vi "Controller Test Bench (10) - Output Not Working.vi"() -> ()   [LabVIEW 2022 SP3]
uses:
  WhiteNoise.ctl
  <vilib>/sound2/lvsound2.llb/Sound Data Format.ctl
  <vilib>/Utility/error.llb/DialogType.ctl
  <vilib>/sound2/lvsound2.llb/Sampling Mode.ctl
  <vilib>/sound2/lvsound2.llb/Sound File Refnum.ctl
  <vilib>/Analysis/4window.llb/windowTd.ctl
  <vilib>/DAQmx/write.llb/DAQmx Write (Analog 1D Wfm NChan NSamp).vi
  <vilib>/DAQmx/read.llb/DAQmx Read (Analog 1D Wfm NChan NSamp).vi
  <vilib>/DAQmx/create/channels.llb/DAQmx Create Channel (AO-Voltage-Basic).vi
  <vilib>/DAQmx/create/channels.llb/DAQmx Create Channel (AI-Acceleration-Accelerometer).vi
  <vilib>/DAQmx/configure/timing.llb/DAQmx Timing (Sample Clock).vi
  <vilib>/sound2/lvsound2.llb/Sound File Info (path).vi
  <vilib>/sound2/lvsound2.llb/Sound File Read Open.vi
  <vilib>/DAQmx/configure/task.llb/DAQmx Configure Logging (TDMS).vi
  <vilib>/sound2/lvsound2.llb/Sound File Read (DBL).vi
  <vilib>/DAQmx/miscellaneous.llb/DAQmx Fill In Error Info.vi
  <vilib>/sound2/lvsound2.llb/Sound Output Set Volume (Single).vi
  <vilib>/sound2/lvsound2.llb/Sound Output Write (DBL).vi
  <vilib>/addons/control/pid/pid.llb/PID (DBL Array).vi
  <vilib>/sound2/lvsound2.llb/Sound Output Write (DBL Single).vi
  <vilib>/measure/maspectr.llb/FFT Spectrum (Mag-Phase) for N Chan.vi
  <vilib>/measure/NI_MAPro.lvlib
  <resource>/objmgr/daqmx.rc
  <vilib>/Analysis/NI_AALPro.lvlib
  <vilib>/measure/NI_MABase.lvlib
  <vilib>/addons/control/pid/NI_PID_pid.lvlib
panel:
  in  "Log Data":bool
  in  "Folder to save file to":path=path "C:/Users/LAV-UFSC/OneDrive - UFSC/Documents/LAV - TCC/Dados-Experimentos/Dados Bancada LABVIEW"
  in  "Display Raw Accel. Readings [m/s^2]":bool=TRUE
  in  "Display Output Signal [V]":bool=TRUE
  out "Output Signal":waveform(dbl)[](graph)
  in  "Number of Samples":i32=41200
  in  "Output Noise":bool=TRUE
  in  "?":T1(tab)=enum."Harmonic"
  in  "number of samples/ch (-1: all)":i32=-1
  in  "Path Sound File":path=path "C:/Users/LAV-UFSC-2023/Documents/LAV-TCC/Dados-Experimentos/Dados Empíricos/Uni - vazio.wav"
  in  "Ganho":i32
  in  "Cluster":T3={"Seed"=0.0, "Standard Deviation"=0.2, "Reset"=FALSE, "Iterator"=1.0} {"Standard Deviation" format="%0.2p"}
  in  "Cluster 2":T4={"Iterator"=1.0, "Waveform Type"=0, "Frequency"=10.0, "Amplitude"=0.25} {"Frequency" format="%0.2p"; "Waveform Type" items=["Sine Wave", "Triangle Wave", "Square Wave", "Sawtooth Wave"]; "Amplitude" format="%0.2p"}
  in  "Active Control":bool
  in  "Tab Control":T5(tab)
  in  "reinitialize? (F)":bool
  out "dt out (s)":dbl format="%.3f"
  in  "setpoint":dbl[](array[numeric])=[0.0] format="%.2f"
  in  "PID gains":T6(array[cluster])=[{"proportional gain (Kc)"=1.0, "integral time (Ti, min)"=0.01, "derivative time (Td, min)"=0.0}] {"derivative time (Td, min)" format="%.3f"; "integral time (Ti, min)" format="%.3f"; "proportional gain (Kc)" format="%.3f"}
  in  "dt (s)":dbl=-1.0 format="%.3f"
  in  "output range":cluster{"output high":dbl, "output low":dbl}[](array[cluster])=[{"output high"=100.0, "output low"=-100.0}] {"output low" format="%.2f"; "output high" format="%.2f"}
  in  "Setpoint":dbl
  in  "Gain":dbl min=0.0 step=0.01
  out "Controller Output Signal":waveform(dbl)[](graph)
  in  "Display Output Control Signal [V]":bool
  out "Actual Sample Rate":dbl=1000.0 format="%0.2f"
  out "Accel.1":waveform(dbl)[](graph)
  out "Accel.2":waveform(dbl)[](graph)
  out "Phase 2":cluster{"f0":dbl, "df":dbl, "phase":dbl[]}[](graph)
  out "Mag 2":cluster{"f0":dbl, "df":dbl, "magnitude":dbl[]}[](graph)
  in  "Show FFT":bool=TRUE
  in  "Save FFT":bool
  in  "Start Reading":bool=TRUE
  in  "Stop":bool
  # "Active Controller"
  # "Output Noise"
  # "Data Acquisition"
  # "RAW - Accel. 1"
  # "FFT - Amplitude"
  # "FFT - Phase"
  # "RAW - Accel. 2"
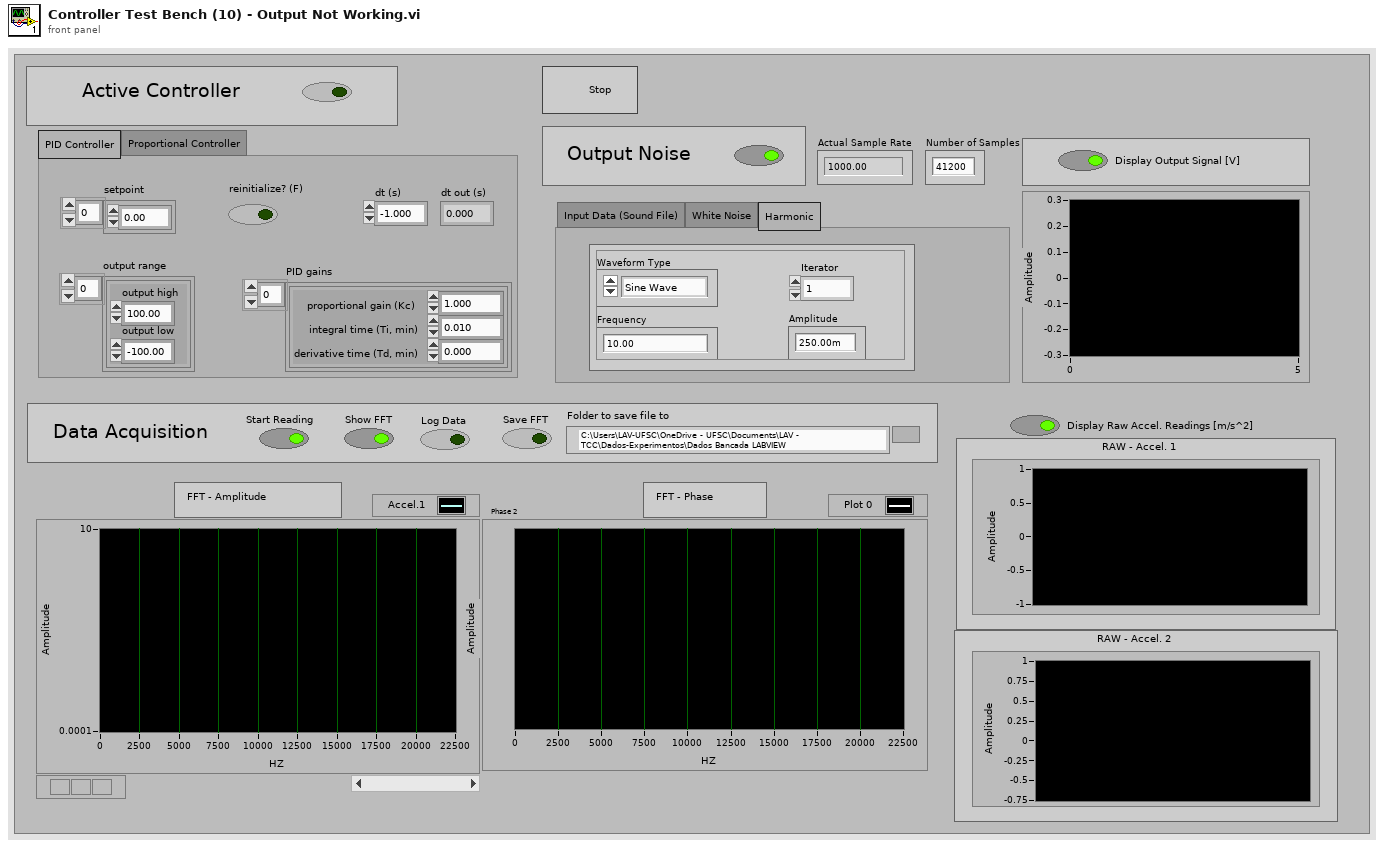
[diagram p1: front panel]
types:
  T1 = enum32{"Input Data (Sound File)", "White Noise", "Harmonic"}
  T2 = typedef "WhiteNoise.ctl" = dbl
  T3 = cluster{"Seed":T2, "Standard Deviation":dbl, "Reset":bool, "Iterator":dbl}
  T4 = cluster{"Iterator":dbl, "Waveform Type":u16, "Frequency":dbl, "Amplitude":dbl}
  T5 = enum32{"PID Controller", "Proportional Controller"}
  T6 = cluster{"proportional gain (Kc)":dbl, "integral time (Ti, min)":dbl, "derivative time (Td, min)":dbl}[]
  T7 = typedef "Sampling Mode.ctl" = i32
  T8 = typedef "DialogType.ctl" = u16
  T9 = typedef "Sound Data Format.ctl" = cluster{"sample rate (S/s)":dbl, "number of channels":i32, "bits per sample":i32}
  T10 = typedef "Sound Output Task ID.ctl" = u32
  T11 = typedef "Sound File Refnum.ctl" = refnum<file>
  T12 = typedef "NI_AALPro.lvlib/windowTd.ctl" = u32
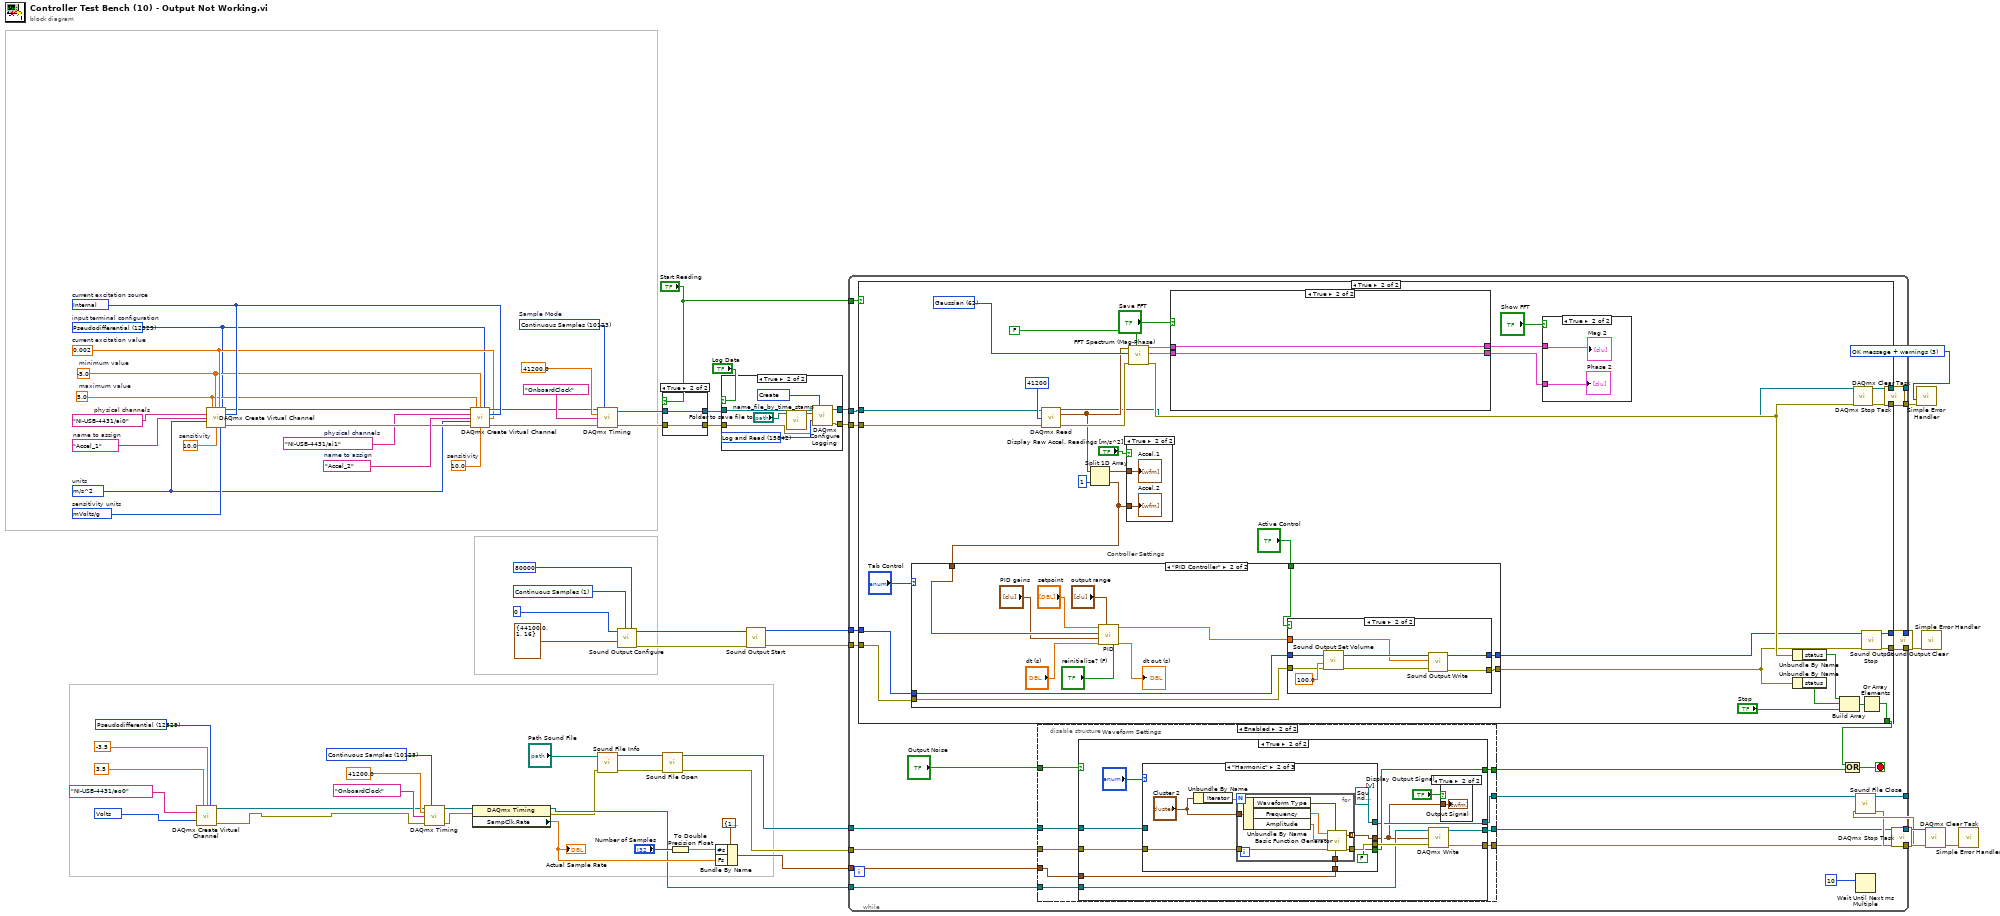
[diagram p0: block diagram]
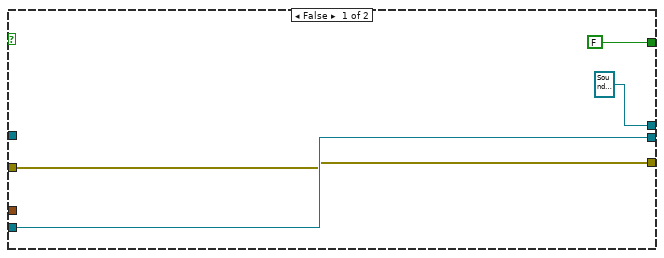
[diagram p5: hidden frame]
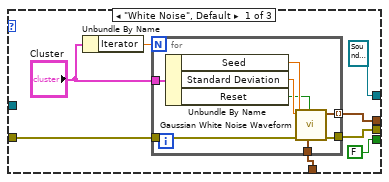
[diagram p7: hidden frame]
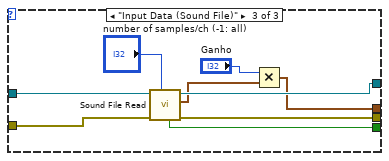
[diagram p8: hidden frame]
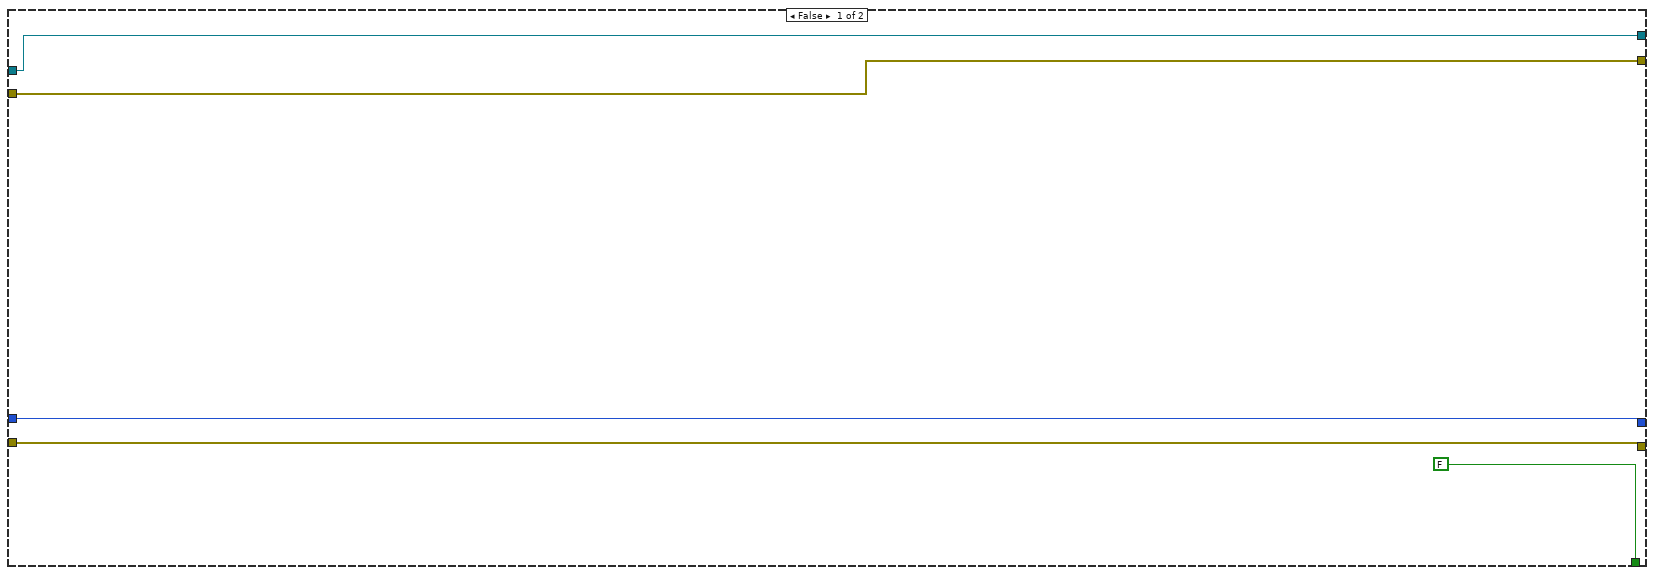
[diagram p9: hidden frame]
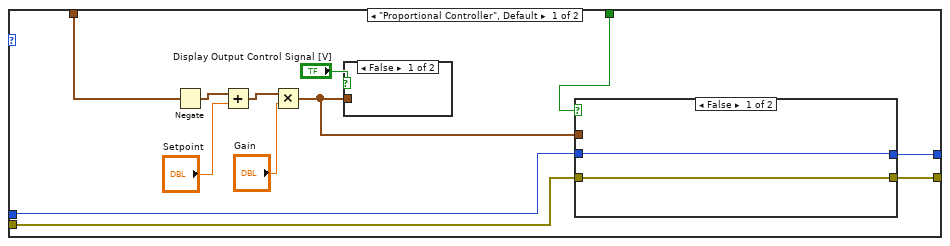
[diagram p11: hidden frame]
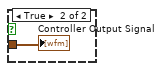
[diagram p12: hidden frame]
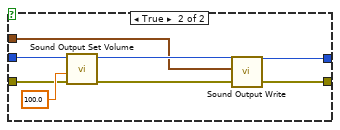
[diagram p13: hidden frame]
diagram:
  w53 = 10123 items=["Finite Samples"=10178, "Continuous Samples"=10123, "Hardware Timed Single Point"=12522] ("sample mode")
  w57 = 12509 items=["mVolts/g"=12509, "Volts/g"=12510]  # sensitivity units
  w58 = 10.0  # sensitivity
  w47 = 0.002  # current excitation value
  w50 = 10200 items=["Internal"=10200, "External"=10167, "None"=10230]  # current excitation source
  w40 = tag "NI-USB-4431/ai0"  # physical channels
  w56 = 10123 items=["Finite Samples"=10178, "Continuous Samples"=10123, "Hardware Timed Single Point"=12522]  # Sample Mode
  w43 = 12529 items=["default"=-1, "RSE"=10083, "NRSE"=10078, "Differential"=10106, "Pseudodifferential"=12529]  # input terminal configuration
  w46 = -5.0  # minimum value
  w45 = 5.0  # maximum value
  w59 = "Accel_1"  # name to assign
  w44 = 12470 items=["g"=10186, "m/s^2"=12470, "in/s^2"=12471, "From Custom Scale"=10065]  # units
  w60 = 10.0  # sensitivity
  w41 = tag "NI-USB-4431/ai1"  # physical channels
  w52 = "Accel_2"  # name to assign
  w61 = T7 1 items=["Finite Samples", "Continuous Samples"] ("sample mode")
  w62 = T8 3 items=["no dialog", "OK message", "continue or stop message", "OK message + warnings", "continue/stop + warnings"] ("type of dialog (OK msg:1)")
  w73 = 12529 items=["Default"=-1, "RSE"=10083, "Differential"=10106, "Pseudodifferential"=12529] ("output terminal configuration")
  w71 = 10348 items=["Volts"=10348, "From Custom Scale"=10065] ("units")
  n1 = call-poly <vilib>:"DAQmx Create Virtual Channel.vi"("maximum value"=3.5, "minimum value"=-3.5, "output terminal configuration"=w73, "physical channels"=tag "NI-USB-4431/ao0", "units"=w71) -> ("task out"=w1:refnum<k21>, "error out"=w2:errorcluster)  [unwired: 9 in]
  n2 = call-poly <vilib>:"DAQmx Create Virtual Channel.vi"("maximum value"=w45, "minimum value"=w46, "input terminal configuration"=w43, "physical channels"=w40, "current excitation source"=w50, "name to assign"=w59, "current excitation value"=w47, "units"=w44, "sensitivity"=w58, "sensitivity units"=w57) -> ("task out"=w42:refnum<k21>, "error out"=w51:errorcluster)  [unwired: 4 in]
  n3 = call-poly <vilib>:"DAQmx Timing.vi"("task/channels in"=w1, "sample mode"=w53, "rate"=41200.0 ("Sample Rate"), "source"=tag "OnboardClock" ("Sample Clock Source"), "error in"=w2) -> ("task out"=w24:refnum<k21>, "error out"=w23:errorcluster)  [unwired: 9 in]
  n4 = call-poly <vilib>:"DAQmx Create Virtual Channel.vi"("task in"=w42, "maximum value"=w45, "minimum value"=w46, "input terminal configuration"=w43, "physical channels"=w41, "current excitation source"=w50, "name to assign"=w52, "current excitation value"=w47, "units"=w44, "error in"=w51, "sensitivity"=w60) -> ("task out"=w49:refnum<k21>, "error out"=w48:errorcluster)  [unwired: 3 in]
  n5 = property class="DAQmx Timing"(reference=w24, error in=w23) -> (reference out=w21:refnum<k21>, error out=w14:errorcluster, "SampClk.Rate"=w25:dbl)
  "Actual Sample Rate" <- w25
  n6 = call-poly <vilib>:"DAQmx Timing.vi"("task/channels in"=w49, "sample mode"=w56, "rate"=41200.0 ("Sample Rate"), "source"=tag "OnboardClock" ("Sample Clock Source"), "error in"=w48) -> ("task out"=w38:refnum<k21>, "error out"=w39:errorcluster)  [unwired: 9 in]
  n7 = call-poly <vilib>:"Sound File Info.vi"("error in (no error)"=w14, "path"="Path Sound File") -> ("error out"=w16:errorcluster, "path out"=w15:path)  [unwired: 6 in, 2 out]
  n8 = call <vilib>:"Sound Output Configure.vi"("number of samples/ch"=80000 ("Number of Samples/ch"), "sample mode"=w61, "sound format"=T9 {"sample rate (S/s)"=44100.0, "number of channels"=1, "bits per sample"=16} ("Sound Format"), "device ID"=u32 0 ("Device ID")) -> ("error out"=w32:errorcluster, "task ID"=w31:T10)  [unwired: 6 in]
  n9 = case shown="True" "Start Reading" {
    tunnel: w39 -> [w79 w81]
    tunnel: w38 -> [w80 w82]
    tunnel: [w80 w82] -> w6
    tunnel: [w79 w81] -> w5
    frame False {
    }
    frame True {
    }
  }
  n10 = call-poly <vilib>:"Sound File Open.vi"("error in (no error)"=w16, "path"=w15) -> ("error out"=w8:errorcluster, "sound file refnum"=w13:T11)  [unwired: 8 in]
  n11 = To Double Precision Float(number="Number of Samples") -> (double precision float=w27:dbl)
  n12 = Bundle By Name(cluster=cluster{"Fs":dbl, "#s":dbl} {"Fs"=1000.0, "#s"=1000.0} ("sampling info"), "#s"=w27, "Fs"=w25) -> (w22:cluster{"Fs":dbl, "#s":dbl})
  n13 = case shown="True" "Log Data" {
    tunnel: w6 -> [w84 w90]
    tunnel: [w84 w89] -> w3
    tunnel: w5 -> [w83 w86]
    tunnel: [w83 w85] -> w4
    frame False {
    }
    frame True {
      w91 = 15848 items=["Open"=10437, "Open or Create"=15846, "Create or Replace"=15847, "Create"=15848] ("operation")
      w92 = 15842 items=["Off"=10231, "Log"=15844, "Log and Read"=15842] ("logging mode")
      n14 = call "name_file_by_time_stamp.vi"("Folder to save file to"="Folder to save file to") -> ("New file path"=w88:path)  [unwired: 10 in]
      n15 = call-poly <vilib>:"DAQmx Configure Logging.vi"("task/channels in"=w90, "operation"=w91, "file path"=w88, "logging mode"=w92, "error in"=w86) -> ("task out"=w89:refnum<k21>, "error out"=w85:errorcluster)  [unwired: 9 in]
    }
  }
  n16 = call <vilib>:"Sound Output Start.vi"("error in (no error)"=w32, "task ID"=w31) -> ("error out"=w29:errorcluster, "task ID out"=w30:T10)  [unwired: 8 in]
  n17 = while {
    tunnel: w3 -> [w113]
    tunnel: w4 -> [w112]
    tunnel: [w110] -> w67
    tunnel: [w111] -> w66
    tunnel: "Start Reading" -> [w109]
    tunnel: [w104] -> w34
    tunnel: [w105] -> w33
    tunnel: w30 -> [w107]
    tunnel: w29 -> [w106]
    tunnel: w8 -> [w102]
    tunnel: w22 -> [w101]
    tunnel: w21 -> [w100]
    tunnel: [w99] -> w11
    tunnel: [w98] -> w18
    tunnel: w13 -> [w97]
    tunnel: [w93] -> w12
    stop <- w95 stop-if-true
    n18 = case shown="True" w109 {
      tunnel: [FALSE w215] -> w96
      tunnel: w113 -> [w185 w186]
      tunnel: w112 -> [w184 w187]
      tunnel: [w185 w188] -> w111
      tunnel: [w184 w203] -> w110
      tunnel: w107 -> [w181 w196]
      tunnel: w106 -> [w182 w195]
      tunnel: [w181 w192] -> w105
      tunnel: [w182 w193] -> w104
      frame False {
      }
      frame True {
        w202 = T12 62 items=["Rectangle"=0, "Hanning"=1, "Hamming"=2, "Blackman-Harris"=3, "Exact Blackman"=4, "Blackman"=5, "Flat Top"=6, "4 Term B-Harris "=7, "7 Term B-Harris"=8, "Low Sidelobe"=9, "Blackman Nuttall"=11, "Triangle"=30, "Bartlett-Hanning"=31, "Bohman"=32, "Parzen"=33, "Welch"=34, "Kaiser"=60, "Dolph-Chebyshev"=61, "Gaussian"=62] ("window")
        # "Controller Settings"
        n19 = call-poly <vilib>:"DAQmx Read.vi"("task/channels in"=w186, "number of samples per channel"=41200, "error in"=w187) -> ("task out"=w188:refnum<k21>, "data"=w199:waveform(dbl)[], "error out"=w204:errorcluster)  [unwired: 10 in]
        n20 = Split 1D Array(array=w199, index=1) -> (first subarray=w189:waveform(dbl)[], second subarray=w190:waveform(dbl)[])
        n21 = case shown="\"PID Controller\"" "Tab Control" {
          tunnel: w190 -> [w225 w252]
          tunnel: w196 -> [w221 w245]
          tunnel: w195 -> [w222 w244]
          tunnel: "Active Control" -> [w220 w243]
          tunnel: [w224 w242] -> w192
          tunnel: [w223 w241] -> w193
          frame "Proportional Controller", Default {
            n22 = Negate(x=w225) -> (-x=w228:waveform(dbl)[])
            n23 = Add(x=w228, y="Setpoint") -> (x+y=w227:waveform(dbl)[])
            n24 = Multiply(x=w227, y="Gain") -> (x*y=w219:waveform(dbl)[])
            n25 = case shown="False" "Display Output Control Signal [V]" {
              tunnel: w219 -> [_ w230]
              frame False {
              }
              frame True {
                "Controller Output Signal" <- w230
              }
            }
            n26 = case shown="False" w220 {
              tunnel: w222 -> [w232 w238]
              tunnel: [w232 w235] -> w223
              tunnel: w221 -> [w231 w239]
              tunnel: [w231 w234] -> w224
              tunnel: w219 -> [_ w233]
              frame False {
              }
              frame True {
                n27 = call-poly <vilib>:"Sound Output Set Volume.vi"("error in (no error)"=w238, "volume"=100.0, "task ID"=w239) -> ("error out"=w236:errorcluster, "task ID out"=w237:T10)  [unwired: 7 in]
                n28 = call-poly <vilib>:"Sound Output Write.vi"("error in (no error)"=w236, "data"=w233, "task ID"=w237) -> ("error out"=w235:errorcluster, "task ID out"=w234:T10)  [unwired: 7 in]
              }
            }
          }
          frame "PID Controller" {
            n29 = call-poly <vilib>:"PID.vi"("reinitialize? (F)"="reinitialize? (F)", "output range"="output range", "dt (s)"="dt (s)", "PID gains"="PID gains", "process variable"=w252, "setpoint"="setpoint") -> ("dt out (s)"=→"dt out (s)":dbl, "output"=w246:dbl[])  [unwired: 4 in]
            n30 = case shown="True" w243 {
              tunnel: w244 -> [w255 w261]
              tunnel: [w255 w258] -> w241
              tunnel: w245 -> [w254 w262]
              tunnel: [w254 w257] -> w242
              tunnel: w246 -> [_ w256]
              frame False {
              }
              frame True {
                n31 = call-poly <vilib>:"Sound Output Set Volume.vi"("error in (no error)"=w261, "volume"=100.0, "task ID"=w262) -> ("error out"=w259:errorcluster, "task ID out"=w260:T10)  [unwired: 7 in]
                n32 = call-poly <vilib>:"Sound Output Write.vi"("error in (no error)"=w259, "data"=w256, "task ID"=w260) -> ("error out"=w258:errorcluster, "task ID out"=w257:T10)  [unwired: 7 in]
              }
            }
          }
        }
        n33 = case shown="True" "Display Raw Accel. Readings [m/s^2]" {
          tunnel: w189 -> [_ w217]
          tunnel: w190 -> [_ w216]
          frame False {
          }
          frame True {
            "Accel.2" <- w216
            "Accel.1" <- w217
          }
        }
        n34 = call-poly <vilib>:"FFT Spectrum (Mag-Phase).vi"("restart averaging (F)"=FALSE, "error in (no error)"=w204, "window"=w202, "time signals"=w199) -> ("error out"=w203:errorcluster, "phases"=w209:cluster{"f0":dbl, "df":dbl, "phase":dbl[]}[], "magnitudes"=w210:cluster{"f0":dbl, "df":dbl, "magnitude":dbl[]}[])  [unwired: 3 in, 2 out]
        n35 = case shown="True" "Save FFT" {
          tunnel: w210 -> [w264 w267]
          tunnel: w209 -> [w265 w266]
          tunnel: [w265 w266] -> w208
          tunnel: [w264 w267] -> w207
          frame False {
          }
          frame True {
          }
        }
        n36 = case shown="True" "Show FFT" {
          tunnel: w207 -> [_ w269]
          tunnel: w208 -> [_ w268]
          frame False {
          }
          frame True {
            "Mag 2" <- w269
            "Phase 2" <- w268
          }
        }
        n37 = Unbundle By Name(w203) -> ("status"=w200:bool)
        n38 = Unbundle By Name(w193) -> ("status"=w206:bool)
        n39 = Build Array(w200, w206, "Stop") -> (w213:bool[])
        n40 = Or Array Elements(Boolean array=w213) -> (logical OR=w215:bool)
      }
    }
    n41 = disable-structure shown="Enabled" {
      disable-tunnel: "Output Noise" -> [_ w118]
      disable-tunnel: w102 -> [_ w119]
      disable-tunnel: w101 -> [_ w117]
      disable-tunnel: w100 -> [_ w120]
      disable-tunnel: [_ w121] -> w99
      disable-tunnel: [_ w122] -> w98
      disable-tunnel: w97 -> [_ w116]
      disable-tunnel: [_ w115] -> w94
      disable-tunnel: [_ w114] -> w93
      frame Disabled {
      }
      frame Enabled {
        # "Waveform Settings"
        n42 = case shown="True" w118 {
          tunnel: [w126 w136] -> w122
          tunnel: [w125 w135] -> w121
          tunnel: w120 -> [w126 w134]
          tunnel: w119 -> [w125 w132]
          tunnel: w117 -> [_ w133]
          tunnel: w116 -> [_ w131]
          tunnel: [FALSE w130] -> w115
          tunnel: [T11 refnum ("sound file refnum out") w129] -> w114
          frame False {
          }
          frame True {
            n43 = case shown="\"Harmonic\"" "?" {
              tunnel: w133 -> [w147 w161 _]
              tunnel: w132 -> [w142 w163 w180]
              tunnel: [w146 w160 w179] -> w137
              tunnel: [w143 w162 w174] -> w128
              tunnel: w131 -> [_ _ w177]
              tunnel: [FALSE FALSE w176] -> w130
              tunnel: [T11 refnum ("sound file refnum out") T11 refnum ("sound file refnum out") w175] -> w129
              frame "White Noise", Default {
                n44 = Unbundle By Name("Cluster") -> ("Iterator"=w145:dbl)
                n45 = for {
                  N: w145 -> [_]
                  tunnel: w142 -> [w155]
                  tunnel: w147 -> [w154]
                  tunnel: [w153] -> w146
                  tunnel: "Cluster" -> [w152]
                  tunnel: [w151] -> w143 mode=indexing
                  n46 = Unbundle By Name(w152) -> ("Seed"=w150:T2, "Standard Deviation"=w149:dbl, "Reset"=w148:bool)
                  n47 = call <vilib>:"Gaussian White Noise Waveform.vi"("sampling info"=w154, "reset signal"=w148, "error in (no error)"=w155, "seed"=w150, "standard deviation"=w149) -> ("error out"=w153:errorcluster, "signal out"=w151:waveform(dbl))  [unwired: 5 in]
                }
              }
              frame "Harmonic" {
                n48 = Unbundle By Name("Cluster 2") -> ("Iterator"=w159:dbl)
                n49 = for {
                  N: w159 -> [_]
                  tunnel: w163 -> [w171]
                  tunnel: w161 -> [w170]
                  tunnel: [w169] -> w160
                  tunnel: "Cluster 2" -> [w168]
                  tunnel: [w164] -> w162 mode=indexing
                  n50 = Unbundle By Name(w168) -> ("Waveform Type"=w167:u16, "Frequency"=w166:dbl, "Amplitude"=w165:dbl)
                  n51 = call <vilib>:"Basic Function Generator.vi"("sampling info"=w170, "signal type"=w167, "error in (no error)"=w171, "amplitude"=w165, "frequency"=w166) -> ("error out"=w169:errorcluster, "signal out"=w164:waveform(dbl))  [unwired: 4 in, 1 out]
                }
              }
              frame "Input Data (Sound File)" {
                n52 = call-poly <vilib>:"Sound File Read.vi"("number of samples/ch (-1: all)"="number of samples/ch (-1: all)", "error in (no error)"=w180, "sound file refnum"=w177) -> ("error out"=w179:errorcluster, "data"=w173:waveform(dbl)[], "sound file refnum out"=w175:T11, "end of file?"=w176:bool)  [unwired: 4 in, 1 out]
                n53 = Multiply(x="Ganho", y=w173) -> (x*y=w174:waveform(dbl)[])
              }
            }
            n54 = call-poly <vilib>:"DAQmx Write.vi"("task/channels in"=w134, "data"=w128, "error in"=w137) -> ("task out"=w136:refnum<k21>, "error out"=w135:errorcluster)  [unwired: 10 in, 1 out]
            n55 = case shown="True" "Display Output Signal [V]" {
              tunnel: w128 -> [_ w139]
              frame False {
              }
              frame True {
                "Output Signal" <- w139
              }
            }
          }
        }
      }
    }
    n56 = Compound Arithmetic op=OR(w96, w94) -> (w95:bool)
    n57 = Wait Until Next ms Multiple(millisecond multiple=u32 10) -> ()  [unwired: 1 out]
  }
  n58 = call <vilib>:"DAQmx Stop Task.vi"("task/channels in"=w66, "error in"=w67) -> ("task out"=w69:refnum<k21>, "error out"=w68:errorcluster)  [unwired: 12 in]
  n59 = call <vilib>:"Sound File Close.vi"("error in (no error)"=w11, "sound file refnum"=w12) -> ("error out"=w10:errorcluster)  [unwired: 9 in]
  n60 = call <vilib>:"Sound Output Stop.vi"("error in (no error)"=w34, "task ID"=w33) -> ("error out"=w37:errorcluster, "task ID out"=w36:T10)  [unwired: 8 in]
  n61 = call <vilib>:"DAQmx Clear Task.vi"("task in"=w69, "error in"=w68) -> ("error out"=w70:errorcluster)  [unwired: 13 in]
  n62 = call <vilib>:"DAQmx Stop Task.vi"("task/channels in"=w18, "error in"=w10) -> ("task out"=w20:refnum<k21>, "error out"=w19:errorcluster)  [unwired: 12 in]
  n63 = call <vilib>:"Sound Output Clear.vi"("error in (no error)"=w37, "task ID"=w36) -> ("error out"=w35:errorcluster)  [unwired: 9 in]
  n64 = call <vilib>:"Simple Error Handler.vi"("type of dialog (OK msg:1)"=w62, "error in (no error)"=w70) -> ()  [unwired: 3 in, 5 out]
  n65 = call <vilib>:"Simple Error Handler.vi"("error in (no error)"=w35) -> ()  [unwired: 4 in, 5 out]
  n66 = call <vilib>:"DAQmx Clear Task.vi"("task in"=w20, "error in"=w19) -> ("error out"=w17:errorcluster)  [unwired: 13 in]
  n67 = call <vilib>:"Simple Error Handler.vi"("error in (no error)"=w17) -> ()  [unwired: 4 in, 5 out]
